vi "niDAQmx Get gRPC Location.vi"(8 "error in":errorcluster) -> (0 "error out":errorcluster, 2 "port":u32, 3 "address":string)   [LabVIEW 2021, in "Session Management niDAQmx.lvlib" / "Session Factory.lvclass"]
doc: "Gets the gRPC Device Server location ofr NI-DAQmx."
uses:
  Session Factory.lvclass
  <vilib>/gRPC/Generated APIs/ni/measurementlink/discovery/v1/RPC Messages/ni_measurementlink_discovery_v1_ResolveServiceRequest.ctl
  Session Factory.lvclass/Session Factory.ctl
  <vilib>/Plug-In SDKs/Clients/Discovery V1/NI Discovery V1 Client.lvlib
  <vilib>/gRPC/Generated APIs/ni/measurementlink/discovery/v1/ni.measurementlink.discovery.v1.api.lvlib
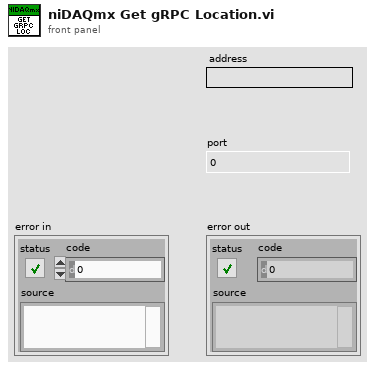
[diagram p1: front panel]
types:
  T1 = typedef "ni.measurementlink.discovery.v1.api.lvlib/ni_measurementlink_discovery_v1_ResolveServiceRequest.ctl" = cluster{"provided_interface":string, "service_class":string, "deployment_target":string, "version":string}
  T2 = typedef "ni.measurementlink.discovery.v1.api.lvlib/ni_measurementlink_discovery_v1_ServiceLocation.ctl" = cluster{"location":string, "insecure_port":string, "ssl_authenticated_port":string}
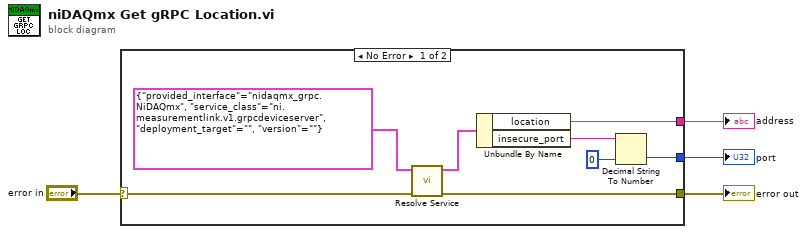
[diagram p0: block diagram]
diagram:
  n1 = case shown="No Error" "error in" {
    selector: "error in" -> [w10 w13]
    tunnel: [w9 w13] -> w3
    tunnel: [w7 _] -> w2
    tunnel: [w6 _] -> w1
    frame No Error {
      n2 = call <vilib>:"Resolve Service.vi"("error in"=w10, "request data"=T1 {"provided_interface"="nidaqmx_grpc.NiDAQmx", "service_class"="ni.measurementlink.v1.grpcdeviceserver", "deployment_target"="", "version"=""}) -> ("error out"=w9:errorcluster, "response data"=w11:T2)  [unwired: 8 in]
      n3 = Unbundle By Name(w11) -> ("location"=w7:string, "insecure_port"=w8:string)
      n4 = Decimal String To Number(string=w8, default (0L)=u32 0 ("default (0 I32)")) -> (number=w6:u32)  [unwired: 1 in, 1 out]
    }
    frame Error {
    }
  }
  "address" <- w2
  "error out" <- w3
  "port" <- w1
